vi "Update Build Constants.vi"(8 "error in (no error)":errorcluster, 11 "Pre-Build Properties":T1) -> (0 "error out":errorcluster, 3 "Pre-Build Properties dup":T1)   [LabVIEW 2013]
uses:
  pre-build properties -- cluster.ctl
  <vilib>/Utility/traverseref.llb/TRef TravTarget.ctl
  <vilib>/Utility/traverseref.llb/VI Scripting - Traverse.lvlib
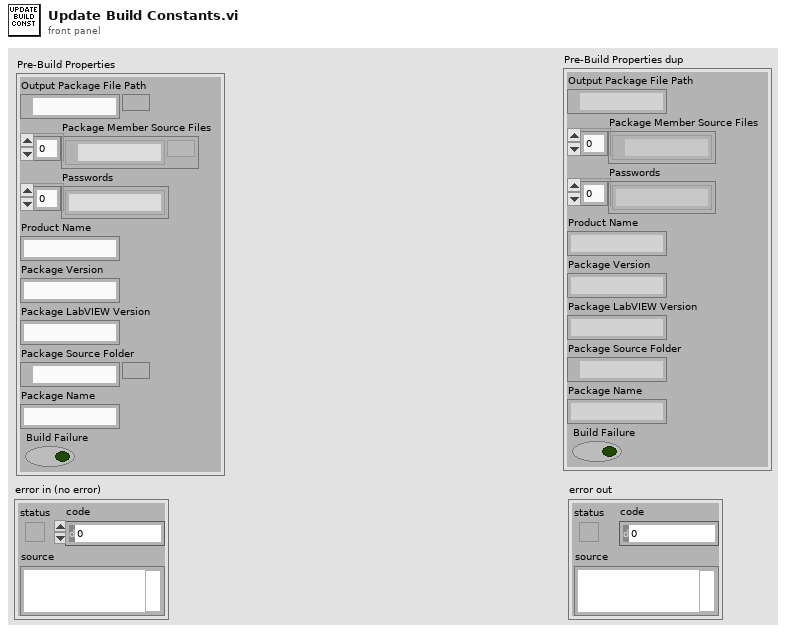
[diagram p1: front panel]
types:
  T1 = typedef "pre-build properties -- cluster.ctl" = cluster{"Output Package File Path":path, "Package Member Source Files":path[], "Passwords":string[], "Product Name":string, "Package Version":string, "Package LabVIEW Version":string, "Package Source Folder":path, "Package Name":string, "Build Failure":bool}
  T2 = typedef "TRef TravTarget.ctl" = enum16{"FP", "BD", "Other"}
  T3 = cluster{"Version String":string, "Name":string, "Copyright":string, "License":string}
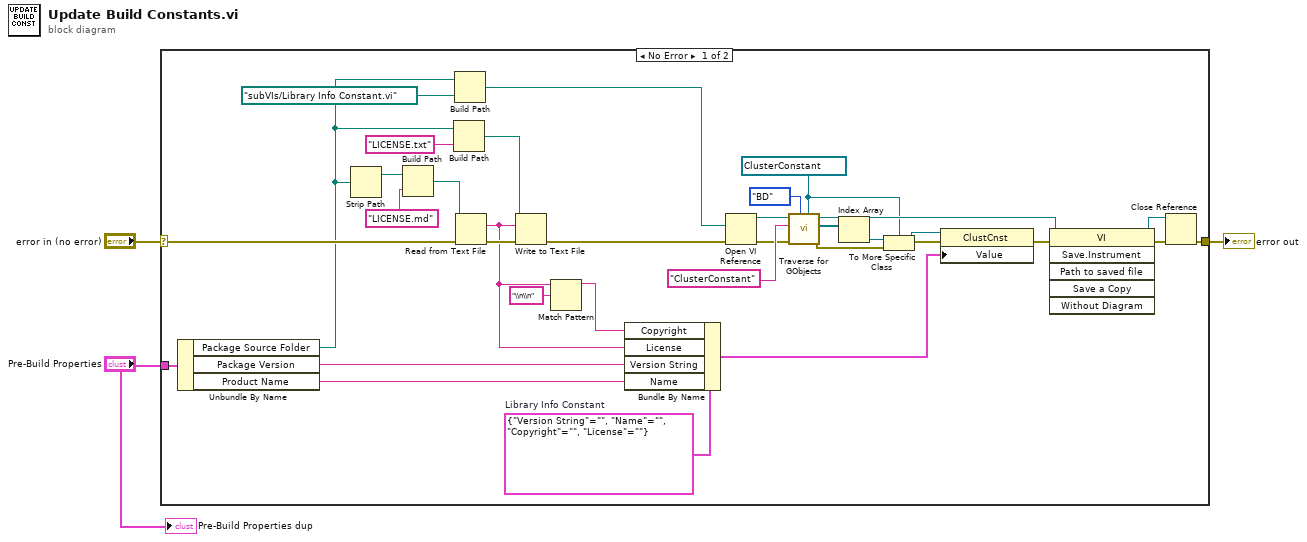
[diagram p0: block diagram]
diagram:
  n1 = case shown="No Error" "error in (no error)" {
    selector: "error in (no error)" -> [w18 w38]
    tunnel: [w36 w38] -> w3
    tunnel: "Pre-Build Properties" -> [w32 _]
    frame No Error {
      w4 = refnum<vi> refnum ("Other Refnum")
      w34 = T3 {"Version String"="", "Name"="", "Copyright"="", "License"=""}  # Library Info Constant
      n2 = Unbundle By Name(w32) -> ("Package Source Folder"=w17:path, "Package Version"=w27:string, "Product Name"=w28:string)
      n3 = Strip Path(path=w17) -> (stripped path=w31:path)  [unwired: 1 out]
      n4 = Build Path(base path=w31, name or relative path="LICENSE.md") -> (appended path=w21:path)
      n5 = Build Path(base path=w17, name or relative path="LICENSE.txt") -> (appended path=w20:path)
      n6 = Build Path(base path=w17, name or relative path=path "subVIs/Library Info Constant.vi" ("base path")) -> (appended path=w33:path)
      n7 = Read from Text File(file (use dialog)=w21, error in=w18) -> (text=w23:string, error out=w25:errorcluster)  [unwired: 2 in, 2 out]
      n8 = Write to Text File(file (use dialog)=w20, text=w23, error in=w25) -> (error out=w24:errorcluster)  [unwired: 1 in, 2 out]
      n9 = Match Pattern(string=w23, regular expression="\\n\\n") -> (before substring=w22:string)  [unwired: 1 in, 3 out]
      n10 = Bundle By Name(cluster=w34, "Copyright"=w22, "License"=w23, "Version String"=w27, "Name"=w28) -> (w10:T3)
      n11 = Open VI Reference(vi path=w33, error in (no error)=w24) -> (vi reference=w16:refnum<vi>, error out=w7:errorcluster)  [unwired: 4 in]
      n12 = call <vilib>:"Traverse for GObjects.vi"("Other Refnum"=w4, "Traverse Target"=TRef_TravTarget."BD", "error in (no error)"=w7, "Class Name"="ClusterConstant", "VI Refnum"=w16) -> ("error out"=w6:errorcluster, "References"=w13:refnum<vi>[], "dup VI Refnum"=w9:refnum<vi>)  [unwired: 3 in, 1 out]
      n13 = Index Array(array=w13) -> (element=w12:refnum<vi>)  [unwired: 1 in]
      n14 = To More Specific Class(target class=w4, reference=w12, error in=w6) -> (specific class reference=w11:refnum<vi>, error out=w5:errorcluster)
      n15 = property class="ClustCnst"(reference=w11, error in=w5, "Value"=w10) -> (error out=w8:errorcluster)  [unwired: 1 out]
      n16 = invoke class="VI" method="Save.Instrument"(reference=w9, error in=w8) -> (reference out=w19:refnum<vi>, error out=w37:errorcluster)  [unwired: 4 in, 4 out]
      n17 = Close Reference(reference=w19, error in (no error)=w37) -> (error out=w36:errorcluster)
    }
    frame Error {
    }
  }
  "error out" <- w3
  "Pre-Build Properties dup" <- "Pre-Build Properties"
